vi "Get FTDI Devices List.vi"() -> (4 "FTDI Serial Numbers":string[](array[string]), 8 "FTDI Serial Ports":string[](array[string]), 10 "FTDI Serial Ports":u32[](array[numeric]))   [LabVIEW 2010]
panel:
  # "Enter values in Write Buffer and run program.  \nWith a loop-back connector, the data is read back into the Read Buffer."
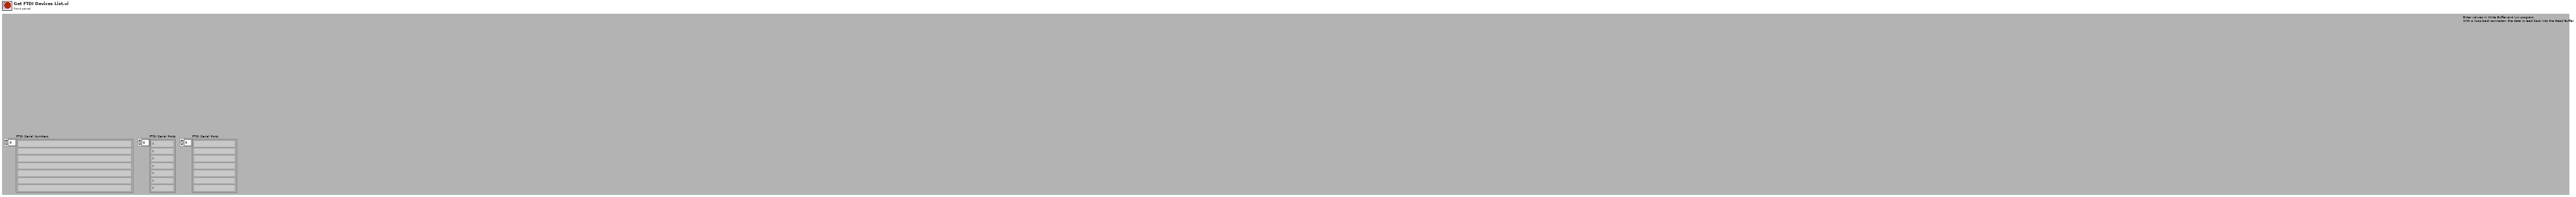
[diagram p1: front panel]
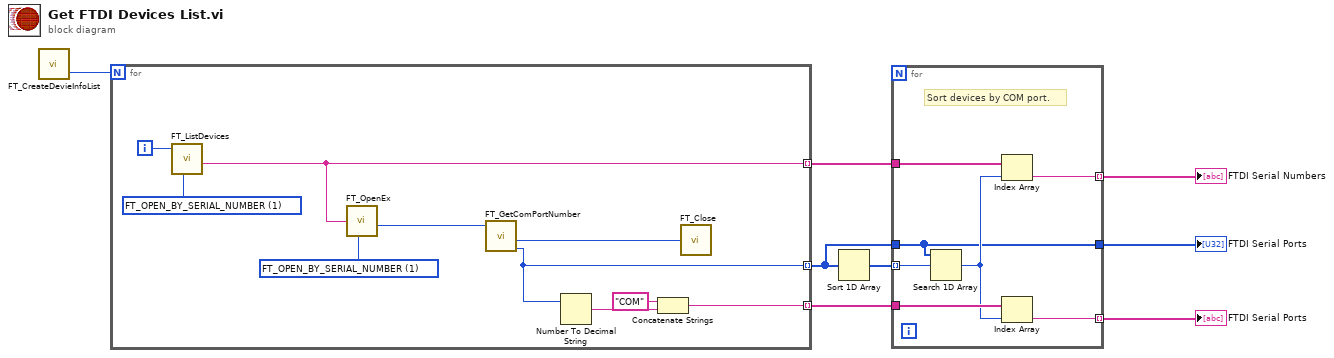
[diagram p0: block diagram]
diagram:
  n1 = call "FT_CreateDevieInfoList.vi"() -> ("lpdwNumDevs"=w8:u32)  [unwired: 2 in, 1 out]
  n2 = for {
    N: w8 -> [_]
    tunnel: [w16] -> w4 mode=indexing
    tunnel: [w10] -> w5 mode=indexing
    tunnel: [w9] -> w6 mode=indexing
    i -> [w18]
    w15 = u32 1 items=["FT_OPEN_BY_SERIAL_NUMBER"=1, "FT_OPEN_BY_DESCRIPTION"=2, "FT_OPEN_BY_LOCATION"=4] ("Flags")
    w17 = u32 1 items=["FT_OPEN_BY_SERIAL_NUMBER"=1, "FT_OPEN_BY_DESCRIPTION"=2, "FT_OPEN_BY_LOCATION"=4] ("Flags")
    n3 = call "FT_ListDevices.vi"("Device Index"=w18, "Flags"=w17) -> ("Device Description"=w16:string)  [unwired: 5 in, 1 out]
    n4 = call "FT_OpenEx.vi"("Device Description"=w16, "Flags"=w15) -> ("Handle"=w14:u32)  [unwired: 5 in, 1 out]
    n5 = call "FT_GetComPortNumber.vi"("Handle"=w14) -> ("Handle"=w13:u32, "ComNumber"=w9:u32)  [unwired: 5 in, 1 out]
    n6 = Number To Decimal String(number=w9) -> (decimal integer string=w11:string)  [unwired: 1 in]
    n7 = Concatenate Strings("COM" ("string"), w11) -> (w10:string)
    n8 = call "FT_Close.vi"("Handle"=w13) -> ()  [unwired: 1 out]
  }
  n9 = Sort 1D Array(array=w6) -> (sorted array=w7:u32[])
  n10 = for {
    tunnel: w7 -> [w25] mode=indexing
    tunnel: w6 -> [w21]
    tunnel: w5 -> [w24]
    tunnel: w4 -> [w23]
    tunnel: [w21] -> w3
    tunnel: [w20] -> w2 mode=indexing
    tunnel: [w19] -> w1 mode=indexing
    # "Sort devices by COM port."
    n11 = Search 1D Array(1D array=w21, element=w25) -> (index of element=w22:i32)  [unwired: 1 in]
    n12 = Index Array(array=w23, index=w22) -> (element=w20:string)
    n13 = Index Array(array=w24, index=w22) -> (element=w19:string)
  }
  "FTDI Serial Numbers" <- w2
  "FTDI Serial Ports" <- w1
  "FTDI Serial Ports" <- w3
